vi "Gui_Fill_Text_From_File.vi"(8 "error in (no error)":errorcluster, 9 "Resource Name":string="Users.txt", 10 "Resource Path":path=path "D:/S.O.F.T.S/LABVIEW/PIL/resources", 11 "Refnum Ch":refnum<vi>) -> (0 "error out":errorcluster, 3 "Refnum Ch out":refnum<vi>)   [LabVIEW 2017]
panel:
  out "Comment out":string
  in  "Comment":string
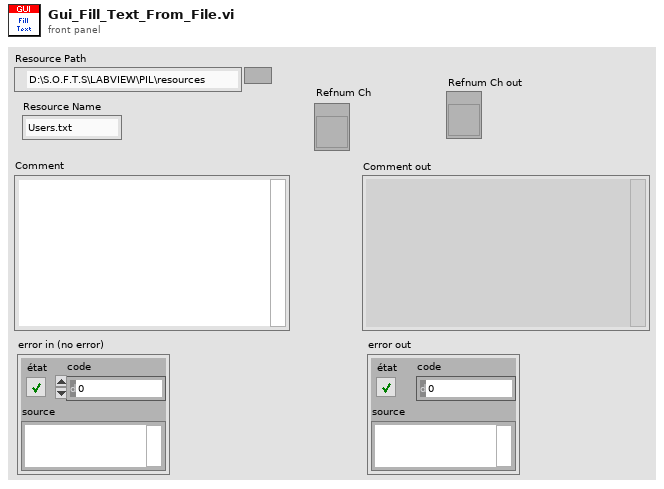
[diagram p1: front panel]
types:
  T1 = enum16{"open", "replace", "create", "open or create", "replace or create", "replace or create with confirmation"}
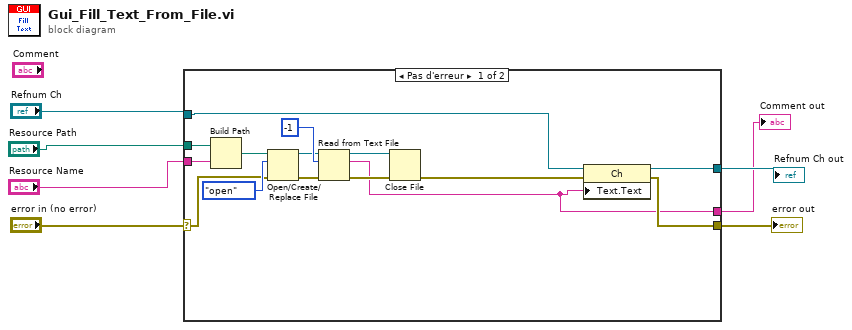
[diagram p0: block diagram]
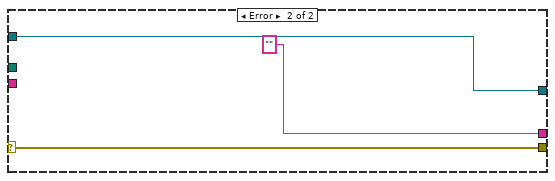
[diagram p2: hidden frame]
diagram:
  n1 = case shown="Pas d'erreur" "error in (no error)" {
    selector: "error in (no error)" -> [w13 w25]
    tunnel: "Resource Path" -> [w22 _]
    tunnel: "Resource Name" -> [w21 _]
    tunnel: [w10 w25] -> w4
    tunnel: "Refnum Ch" -> [w12 w24]
    tunnel: [w9 w24] -> w2
    tunnel: [w8 ""] -> w1
    frame No Error {
      n2 = Build Path(base path=w22, name or relative path=w21) -> (appended path=w18:path)
      n3 = Open/Create/Replace File ("Ouvrir/Créer/Remplacer un fichier")(file path (use dialog)=w18, error in=w13, operation (0:open)=T1."open") -> (refnum out=w19:refnum<file>, error out=w16:errorcluster)  [unwired: 3 in, 1 out]
      n4 = Read from Text File ("Lire un fichier texte")(file (use dialog)=w19, count=-1 ("nombre"), error in=w16) -> (refnum out=w14:refnum<file>, text=w8:string, error out=w15:errorcluster)  [unwired: 1 in, 1 out]
      n5 = Close File(refnum=w14, error in=w15) -> (error out=w11:errorcluster)  [unwired: 1 out]
      n6 = property class="Ch"(reference=w12, error in=w11, "Text.Text"=w8) -> (reference out=w9:refnum<vi>, error out=w10:errorcluster)
    }
    frame Error {
    }
  }
  "error out" <- w4
  "Refnum Ch out" <- w2
  "Comment out" <- w1
